vi "GetStatus.vi"(8 "error in (no error)":errorcluster, 11 "S4ACS_GUI in":refnum<class "S4ACS_GUI.lvclass">) -> (0 "error out":errorcluster, 1 "output cluster":T1, 3 "S4ACS_GUI out":refnum<class "S4ACS_GUI.lvclass">)   [LabVIEW 2018, in "S4ACS_GUI.lvclass"]
uses:
  S4ACS_GUI.lvclass
  S4ACS_GUI.lvclass/S4ACS_GUI.ctl
  Instrument/Instrument.lvclass/Instrument.ctl
  Device/Optics/Optics.lvclass/Optics.ctl
  Device/Optics/Opt_Selector/Opt_Selector.lvclass
  C:/Users/observer/Desktop/Sparc4GUI/SPARC4_GUI/Device/Optics/Optics.lvclass
  Device/Optics/Opt_Continuous/Opt_Continuous.lvclass
  SyncBox/Sync Box.lvclass
  Acquisition/Acquisition.lvclass
  Channel/Channel.lvclass
  Interface/Interface.lvclass
  Trigger/Trigger.lvclass
  Device/Optics/Optics.lvclass
  Instrument/Instrument.lvclass
panel:
  in  "Cluster":T1
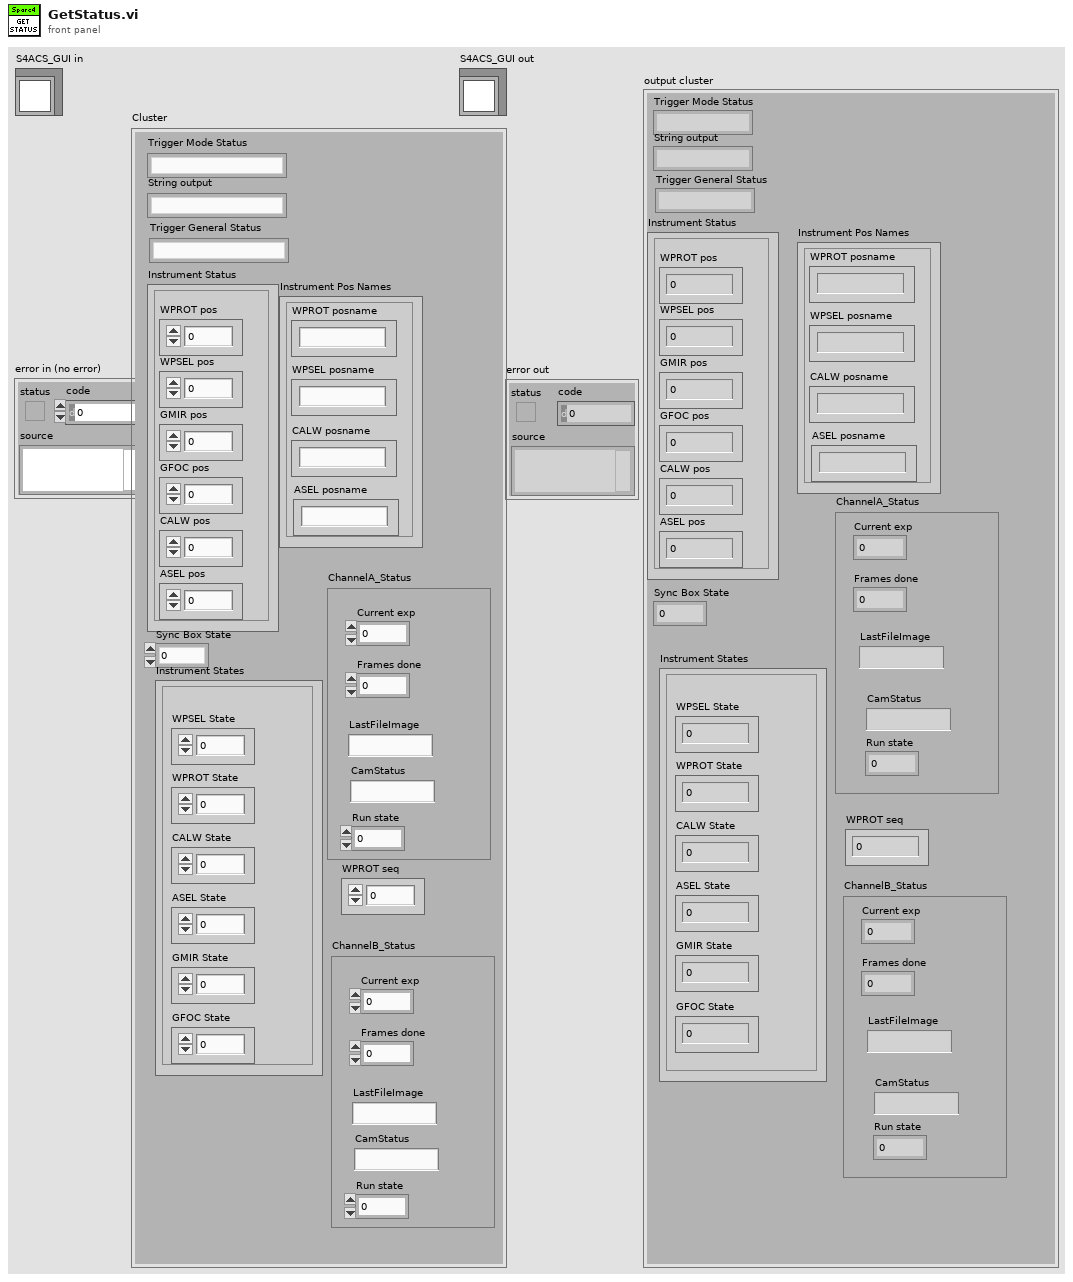
[diagram p1: front panel]
types:
  T1 = cluster{"Trigger Mode Status":string, "String output":string, "Instrument Status":cluster{"WPROT pos":dbl, "WPSEL pos":dbl, "GMIR pos":dbl, "GFOC pos":dbl, "CALW pos":dbl, "ASEL pos":dbl}, "Sync Box State":i32, "Trigger General Status":string, "Instrument States":cluster{"WPSEL State":i32, "WPROT State":i32, "CALW State":i32, "ASEL State":i32, "GMIR State":i32, "GFOC State":i32}, "Instrument Pos Names":cluster{"WPROT posname":string, "WPSEL posname":string, "CALW posname":string, "ASEL posname":string}, "ChannelA_Status":cluster{"Current exp":dbl, "Frames done":u32, "LastFileImage":string, "CamStatus":string, "Run state":u32}, "WPROT seq":u16, "ChannelB_Status":cluster{"Current exp":dbl, "Frames done":u32, "LastFileImage":string, "CamStatus":string, "Run state":u32}}
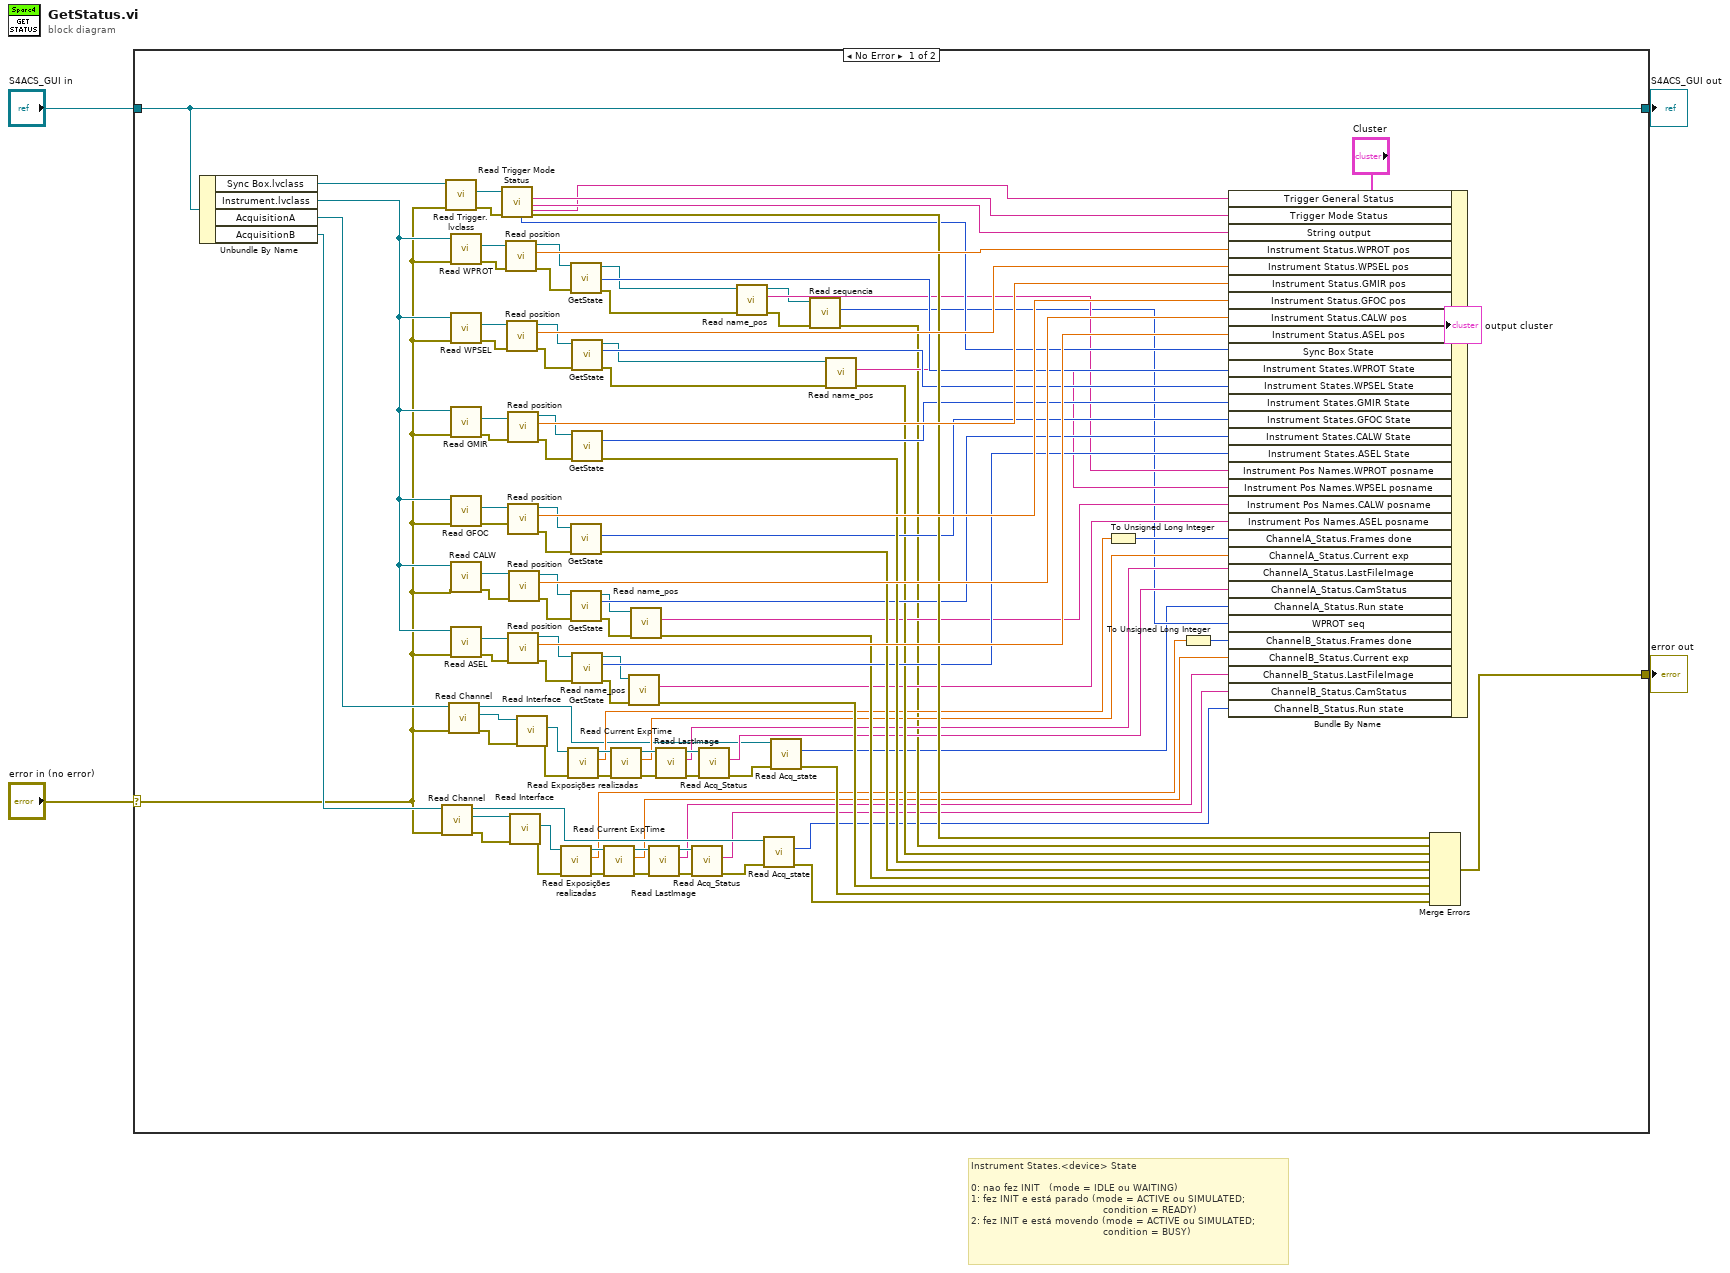
[diagram p0: block diagram]
diagram:
  # "Instrument States.<device> State\n\n0: nao fez INIT   (mode = IDLE ou WAITING)\n1: fez INIT e está parado (mode = ACTIVE ou SIMULATED;\n                                            condition = READY)\n2: fez INIT e está movendo (mode = ACTIVE ou SIMULATED;\n                                            condition = BUSY)"
  n1 = case shown="No Error" "error in (no error)" {
    selector: "error in (no error)" -> [w12 w117]
    tunnel: [w88 w117] -> w3
    tunnel: [w115 w116] -> w1
    tunnel: "S4ACS_GUI in" -> [w115 w116]
    frame No Error {
      n2 = Unbundle By Name(w115) -> ("Sync Box.lvclass"=w114:refnum<class "Sync Box.lvclass">, "Instrument.lvclass"=w108:refnum<class "Instrument.lvclass">, "AcquisitionA"=w49:refnum<class "Acquisition.lvclass">, "AcquisitionB"=w15:refnum<class "Acquisition.lvclass">)
      n3 = call-dynamic "Read Channel.vi"("error in (no error)"=w12, "Acquisition in"=w15) -> ("error out"=w16:errorcluster, "Channel.lvclass"=w14:refnum<class "Channel.lvclass">, "Acquisition out"=w13:refnum<class "Acquisition.lvclass">)  [unwired: 7 in]
      n4 = call-dynamic "Read Trigger.lvclass.vi"("error in (no error)"=w12, "Sync Box in"=w114) -> ("error out"=w87:errorcluster, "Trigger.lvclass"=w113:refnum<class "Trigger.lvclass">)  [unwired: 7 in, 1 out]
      n5 = call-dynamic "Read Channel.vi"("error in (no error)"=w12, "Acquisition in"=w49) -> ("error out"=w47:errorcluster, "Channel.lvclass"=w48:refnum<class "Channel.lvclass">, "Acquisition out"=w26:refnum<class "Acquisition.lvclass">)  [unwired: 7 in]
      n6 = call "Read WPROT.vi"("error in (no error)"=w12, "Instrument in"=w108) -> ("error out"=w105:errorcluster, "Opt_Selector.lvclass"=w106:refnum<class "Opt_Selector.lvclass">)  [unwired: 7 in, 1 out]
      n7 = call "Read WPSEL.vi"("error in (no error)"=w12, "Instrument in"=w108) -> ("error out"=w107:errorcluster, "Opt_Selector.lvclass"=w104:refnum<class "Opt_Selector.lvclass">)  [unwired: 7 in, 1 out]
      n8 = call "Read GMIR.vi"("error in (no error)"=w12, "Instrument in"=w108) -> ("error out"=w103:errorcluster, "Opt_Continuous.lvclass"=w101:refnum<class "Opt_Continuous.lvclass">)  [unwired: 7 in, 1 out]
      n9 = call "Read GFOC.vi"("error in (no error)"=w12, "Instrument in"=w108) -> ("error out"=w99:errorcluster, "Opt_Continuous.lvclass"=w100:refnum<class "Opt_Continuous.lvclass">)  [unwired: 7 in, 1 out]
      n10 = call "Read CALW.vi"("error in (no error)"=w12, "Instrument in"=w108) -> ("error out"=w102:errorcluster, "Opt_Selector.lvclass"=w98:refnum<class "Opt_Selector.lvclass">)  [unwired: 7 in, 1 out]
      n11 = call "Read ASEL.vi"("error in (no error)"=w12, "Instrument in"=w108) -> ("error out"=w97:errorcluster, "Opt_Selector.lvclass"=w96:refnum<class "Opt_Selector.lvclass">)  [unwired: 7 in, 1 out]
      n12 = call-dynamic "Read Trigger Mode Status.vi"("error in (no error)"=w87, "Trigger in"=w113) -> ("error out"=w89:errorcluster, "String output"=w109:string, "Trigger Mode Status"=w111:string, "State"=w86:i32, "Trigger General Status"=w85:string)  [unwired: 4 in, 1 out]
      n13 = call "Read position.vi"("error in (no error)"=w105, "Optics in"=w106) -> ("error out"=w83:errorcluster, "position"=w95:dbl, "Optics out"=w84:refnum<class "Opt_Selector.lvclass">)  [unwired: 7 in]
      n14 = call "Read position.vi"("error in (no error)"=w107, "Optics in"=w104) -> ("error out"=w80:errorcluster, "position"=w94:dbl, "Optics out"=w81:refnum<class "Opt_Selector.lvclass">)  [unwired: 7 in]
      n15 = call "Read position.vi"("error in (no error)"=w103, "Optics in"=w101) -> ("error out"=w77:errorcluster, "position"=w93:dbl, "Optics out"=w78:refnum<class "Opt_Continuous.lvclass">)  [unwired: 7 in]
      n16 = call "Read position.vi"("error in (no error)"=w99, "Optics in"=w100) -> ("error out"=w73:errorcluster, "position"=w92:dbl, "Optics out"=w74:refnum<class "Opt_Continuous.lvclass">)  [unwired: 7 in]
      n17 = call "Read position.vi"("error in (no error)"=w97, "Optics in"=w96) -> ("error out"=w66:errorcluster, "position"=w90:dbl, "Optics out"=w67:refnum<class "Opt_Selector.lvclass">)  [unwired: 7 in]
      n18 = call "Read position.vi"("error in (no error)"=w102, "Optics in"=w98) -> ("error out"=w69:errorcluster, "position"=w91:dbl, "Optics out"=w70:refnum<class "Opt_Selector.lvclass">)  [unwired: 7 in]
      n19 = call-dynamic "Read Interface.vi"("error in (no error)"=w16, "Channel in"=w14) -> ("error out"=w21:errorcluster, "Interface.lvclass"=w17:refnum<class "Interface.lvclass">)  [unwired: 7 in, 1 out]
      n20 = call-dynamic "Read Interface.vi"("error in (no error)"=w47, "Channel in"=w48) -> ("error out"=w37:errorcluster, "Interface.lvclass"=w46:refnum<class "Interface.lvclass">)  [unwired: 7 in, 1 out]
      n21 = call-dynamic "Read Exposições realizadas.vi"("error in (no error)"=w21, "Interface in"=w17) -> ("error out"=w22:errorcluster, "Exposições realizadas"=w10:dbl, "Interface out"=w18:refnum<class "Interface.lvclass">)  [unwired: 7 in]
      n22 = call-dynamic "Read Exposições realizadas.vi"("error in (no error)"=w37, "Interface in"=w46) -> ("error out"=w36:errorcluster, "Exposições realizadas"=w41:dbl, "Interface out"=w45:refnum<class "Interface.lvclass">)  [unwired: 7 in]
      n23 = call-dynamic "GetState.vi"("error in (no error)"=w83, "Optics in"=w84) -> ("error out"=w64:errorcluster, "state"=w82:i32, "Optics out"=w63:refnum<class "Opt_Selector.lvclass">)  [unwired: 7 in]
      n24 = call-dynamic "GetState.vi"("error in (no error)"=w73, "Optics in"=w74) -> ("error out"=w72:errorcluster, "state"=w71:i32)  [unwired: 7 in, 1 out]
      n25 = call-dynamic "GetState.vi"("error in (no error)"=w69, "Optics in"=w70) -> ("error out"=w57:errorcluster, "state"=w68:i32, "Optics out"=w55:refnum<class "Opt_Selector.lvclass">)  [unwired: 7 in]
      n26 = call-dynamic "GetState.vi"("error in (no error)"=w80, "Optics in"=w81) -> ("error out"=w60:errorcluster, "state"=w79:i32, "Optics out"=w59:refnum<class "Opt_Selector.lvclass">)  [unwired: 7 in]
      n27 = call-dynamic "GetState.vi"("error in (no error)"=w77, "Optics in"=w78) -> ("error out"=w76:errorcluster, "state"=w75:i32)  [unwired: 7 in, 1 out]
      n28 = call-dynamic "GetState.vi"("error in (no error)"=w66, "Optics in"=w67) -> ("error out"=w53:errorcluster, "state"=w65:i32, "Optics out"=w51:refnum<class "Opt_Selector.lvclass">)  [unwired: 7 in]
      n29 = call-dynamic "Read Current ExpTime.vi"("error in (no error)"=w22, "Interface in"=w18) -> ("error out"=w23:errorcluster, "Current ExpTime"=w8:dbl, "Interface out"=w19:refnum<class "Interface.lvclass">)  [unwired: 7 in]
      n30 = call-dynamic "Read Current ExpTime.vi"("error in (no error)"=w36, "Interface in"=w45) -> ("error out"=w35:errorcluster, "Current ExpTime"=w42:dbl, "Interface out"=w44:refnum<class "Interface.lvclass">)  [unwired: 7 in]
      n31 = call "Read name_pos.vi"("error in (no error)"=w53, "Optics in"=w51) -> ("error out"=w52:errorcluster, "name_pos"=w50:string)  [unwired: 7 in, 1 out]
      n32 = call "Read name_pos.vi"("error in (no error)"=w57, "Optics in"=w55) -> ("error out"=w56:errorcluster, "name_pos"=w54:string)  [unwired: 7 in, 1 out]
      n33 = call-dynamic "Read LastImage.vi"("error in (no error)"=w23, "Interface in"=w19) -> ("error out"=w24:errorcluster, "LastImage"=w7:string, "Interface out"=w20:refnum<class "Interface.lvclass">)  [unwired: 7 in]
      n34 = call-dynamic "Read LastImage.vi"("error in (no error)"=w35, "Interface in"=w44) -> ("error out"=w34:errorcluster, "LastImage"=w39:string, "Interface out"=w43:refnum<class "Interface.lvclass">)  [unwired: 7 in]
      n35 = call-dynamic "Read Acq_Status.vi"("error in (no error)"=w24, "Interface in"=w20) -> ("error out"=w25:errorcluster, "Acq_Status"=w6:string)  [unwired: 7 in, 1 out]
      n36 = call-dynamic "Read Acq_Status.vi"("error in (no error)"=w34, "Interface in"=w43) -> ("error out"=w27:errorcluster, "Acq_Status"=w38:string)  [unwired: 7 in, 1 out]
      n37 = call "Read name_pos.vi"("error in (no error)"=w64, "Optics in"=w63) -> ("error out"=w32:errorcluster, "name_pos"=w62:string, "Optics out"=w33:refnum<class "Opt_Selector.lvclass">)  [unwired: 7 in]
      n38 = call-dynamic "Read Acq_state.vi"("error in (no error)"=w25, "Acquisition in"=w13) -> ("error out"=w11:errorcluster, "Acq_state"=w5:u32)  [unwired: 7 in, 1 out]
      n39 = call-dynamic "Read Acq_state.vi"("error in (no error)"=w27, "Acquisition in"=w26) -> ("error out"=w28:errorcluster, "Acq_state"=w29:u32)  [unwired: 7 in, 1 out]
      n40 = call-dynamic "Read sequencia.vi"("error in (no error)"=w32, "Opt_Selector in"=w33) -> ("error out"=w31:errorcluster, "sequencia"=w30:u16)  [unwired: 7 in, 1 out]
      n41 = call "Read name_pos.vi"("error in (no error)"=w60, "Optics in"=w59) -> ("error out"=w61:errorcluster, "name_pos"=w58:string)  [unwired: 7 in, 1 out]
      n42 = To Unsigned Long Integer(number=w41) -> (unsigned 32bit integer=w40:u32)
      n43 = To Unsigned Long Integer(number=w10) -> (unsigned 32bit integer=w9:u32)
      n44 = Bundle By Name(cluster="Cluster", "Trigger General Status"=w85, "Trigger Mode Status"=w111, "String output"=w109, "Instrument Status.WPROT pos"=w95, "Instrument Status.WPSEL pos"=w94, "Instrument Status.GMIR pos"=w93, "Instrument Status.GFOC pos"=w92, "Instrument Status.CALW pos"=w91, "Instrument Status.ASEL pos"=w90, "Sync Box State"=w86, "Instrument States.WPROT State"=w82, "Instrument States.WPSEL State"=w79, "Instrument States.GMIR State"=w75, "Instrument States.GFOC State"=w71, "Instrument States.CALW State"=w68, "Instrument States.ASEL State"=w65, "Instrument Pos Names.WPROT posname"=w62, "Instrument Pos Names.WPSEL posname"=w58, "Instrument Pos Names.CALW posname"=w54, "Instrument Pos Names.ASEL posname"=w50, "ChannelA_Status.Frames done"=w40, "ChannelA_Status.Current exp"=w42, "ChannelA_Status.LastFileImage"=w39, "ChannelA_Status.CamStatus"=w38, "ChannelA_Status.Run state"=w29, "WPROT seq"=w30, "ChannelB_Status.Frames done"=w9, "ChannelB_Status.Current exp"=w8, "ChannelB_Status.LastFileImage"=w7, "ChannelB_Status.CamStatus"=w6, "ChannelB_Status.Run state"=w5) -> (→"output cluster":T1)
      n45 = Merge Errors(w89, w31, w61, w76, w72, w56, w52, w28, w11) -> (w88:errorcluster)
    }
    frame Error {
    }
  }
  "error out" <- w3
  "S4ACS_GUI out" <- w1
